vi "Dispose.vi"(8 "error in (no error)":errorcluster, 11 "BombedWall":refnum<class "BombedWall.lvclass">) -> (0 "error out":errorcluster)   [LabVIEW 2020]
uses:
  BombedWall.lvclass
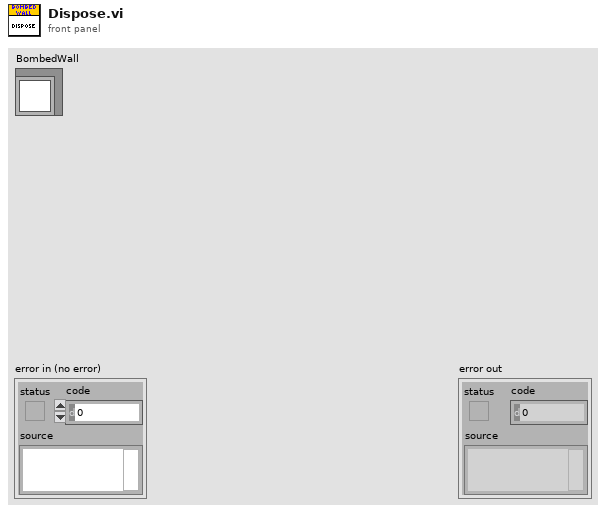
[diagram p1: front panel]
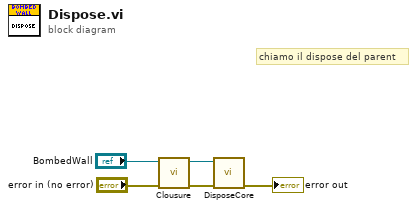
[diagram p0: block diagram]
diagram:
  # "chiamo il dispose del parent"
  n1 = call-dynamic "Clousure.vi"("error in (no error)"="error in (no error)", "BombedWall"="BombedWall") -> ("error out"=w4:errorcluster, "BombedWall"=w3:refnum<class "BombedWall.lvclass">)  [unwired: 8 in]
  n2 = call-dynamic "DisposeCore.vi"("error in (no error)"=w4, "BombedWall"=w3) -> ("error out"=→"error out":errorcluster)  [unwired: 8 in, 1 out]
